vi "Digital Patterns Page.vi"(8 "error in (no error)":errorcluster, 11 "Node Ptr":T1 format="%.0x") -> (0 "error out":errorcluster)   [LabVIEW 2020, in "Engine Simulation Toolkit System Explorer.lvlib"]
uses:
  Engine Simulation Toolkit System Explorer.lvlib
  <vilib>/NI VeriStand/Custom Device API/Custom Device Item Ref.ctl
  Digital Patterns Page Data.ctl
  Digital Pattern.ctl
  Digital Pattern Base.ctl
  Digital Pattern Remove Edge.ctl
  Digital Pattern Add Pulse.ctl
  File Formats.lvlibp/Parent/EST Pattern.ctl
  Shared/Constants and GUIDs.vi
  Shared/Properties.vi
  <vilib>/NI VeriStand/Custom Device API/Custom Device API.lvlib
  Shared/Engine Simulation Toolkit Shared.lvlib
  <vilib>/NI/GXML/GXML.lvlib
  File Formats.lvlibp/Parent/FileFormat.lvclass
panel:
  in  "FPGA Resource":u16(ring) items=["Select an item..."]
  in  "pattern_remove":bool
  in  "pattern_add":bool caption="remove_add"
  in  "add_add":bool caption="remove_add"
  in  "Chart_Offset":dbl caption="Offset" format="%#_6f"
  in  "Chart_Tooth":u16 caption="Tooth"
  in  "Chart_Position":dbl caption="Position" format="%#_6f"
  in  "Edge":bool
  in  "remove_Tooth":u16 caption="Start\nTooth"
  in  "add_Offset":dbl caption="Offset"
  in  "add_Width":dbl caption="Width"
  in  "add_Tooth":u16 caption="Tooth"
  in  "base_Offset":dbl caption="Offset"
  in  "base_Toothwidth":dbl caption="Tooth width"
  in  "base_teeth":u16 caption="Teeth"
  in  "base_Length":dbl caption="Length"
  in  "add_remove":bool
  in  "remove_remove":bool
  in  "remove_add":bool
  in  "Pattern Name":string caption="Name"
  in  "Edges Removed":i32(listbox)
  in  "Pulses Added":i32(listbox)
  in  "Patterns":i32[](listbox)
  in  "Zoom":cluster{dbl, dbl}(slide)={360.0, -360.0} scale=-360.0..360.0
  out "Pattern Plot":cluster{dbl[], dbl[]}[](graph)
  in  "Header":cluster{"Section Name":string}={"Section Name"="Digital Patterns Settings"}
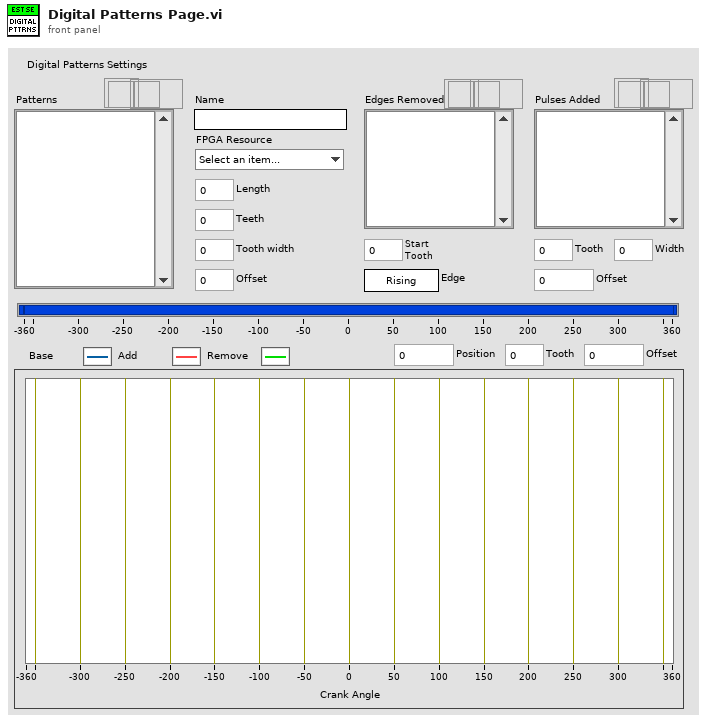
[diagram p1: front panel]
types:
  T1 = typedef "Custom Device API.lvlib/Custom Device Item Ref.ctl" = u64
  T2 = typedef "Engine Simulation Toolkit System Explorer.lvlib/Digital Patterns Page Data.ctl" = cluster{"SysExp Event":refnum<event-registration>, "Init done":bool, "Node Ptr":T1, "Ctrl Refs":cluster{"Header":refnum<vi>, "Pattern Plot":refnum<vi>, "Zoom":refnum<vi>, "Select Pattern":refnum<vi>, "Add List":refnum<vi>, "Remove List":refnum<vi>, "Pattern Name":refnum<vi>, "remove_add":refnum<vi>, "remove_remove":refnum<vi>, "add_remove":refnum<vi>, "base_Length":refnum<vi>, "base_teeth":refnum<vi>, "base_Toothwidth":refnum<vi>, "base_Offset":refnum<vi>, "add_Tooth":refnum<vi>, "add_Width":refnum<vi>, "add_Offset":refnum<vi>, "remove_Tooth":refnum<vi>, "remove_Edge":refnum<vi>, "Chart_Position":refnum<vi>, "Chart_Tooth":refnum<vi>, "Chart_Offset":refnum<vi>, "add_add":refnum<vi>, "pattern_remove":refnum<vi>, "pattern_add":refnum<vi>, "FPGA Resource":refnum<vi>}, "SE ref":refnum<vi>, "Patterns":T3[], "Sel patterns":i32[], "rotations":u16, "Need save":bool, "Rem List":i32, "Add List":i32, "FPGA Resources":string[]}
  T3 = typedef "Engine Simulation Toolkit System Explorer.lvlib/Digital Pattern.ctl" = cluster{"Name":string, "Base":T4, "Remove":T5[], "Add":T6[], "FPGA Resource":string}
  T4 = typedef "Engine Simulation Toolkit System Explorer.lvlib/Digital Pattern Base.ctl" = cluster{"Length":dbl, "Teeth":u16, "Width":dbl, "Offset":dbl}
  T5 = typedef "Engine Simulation Toolkit System Explorer.lvlib/Digital Pattern Remove Edge.ctl" = cluster{"Tooth":u16, "Edge":bool}
  T6 = typedef "Engine Simulation Toolkit System Explorer.lvlib/Digital Pattern Add Pulse.ctl" = cluster{"Tooth":u16, "Offset":dbl, "Width":dbl}
  T7 = typedef "Custom Device API.lvlib/Custom Device Commands.ctl" = enum16{"Default", "Item renamed", "Shutdown", "Dynamic button pressed"}
  T8 = typedef "LVPoint32TypeDef.ctl" = cluster{"Horizontal":i32, "Vertical":i32}
  T9 = typedef "File Formats.lvlibp/FileFormat.lvclass/EST Pattern.ctl" = cluster{"Base":cluster{"Length":dbl, "Teeth":u16, "Width":dbl, "Offset":dbl}, "Remove":cluster{"Tooth":u16, "Edge":bool}[], "Add":cluster{"Tooth":u16, "Offset":dbl, "Width":dbl}[]}
  T10 = cluster{"Length":dbl, "Teeth":u16, "Width":dbl, "Offset":dbl}
  T11 = cluster{"Tooth":u16, "Offset":dbl, "Width":dbl}[]
  T12 = cluster{"ip list property name":string, string[]}[]
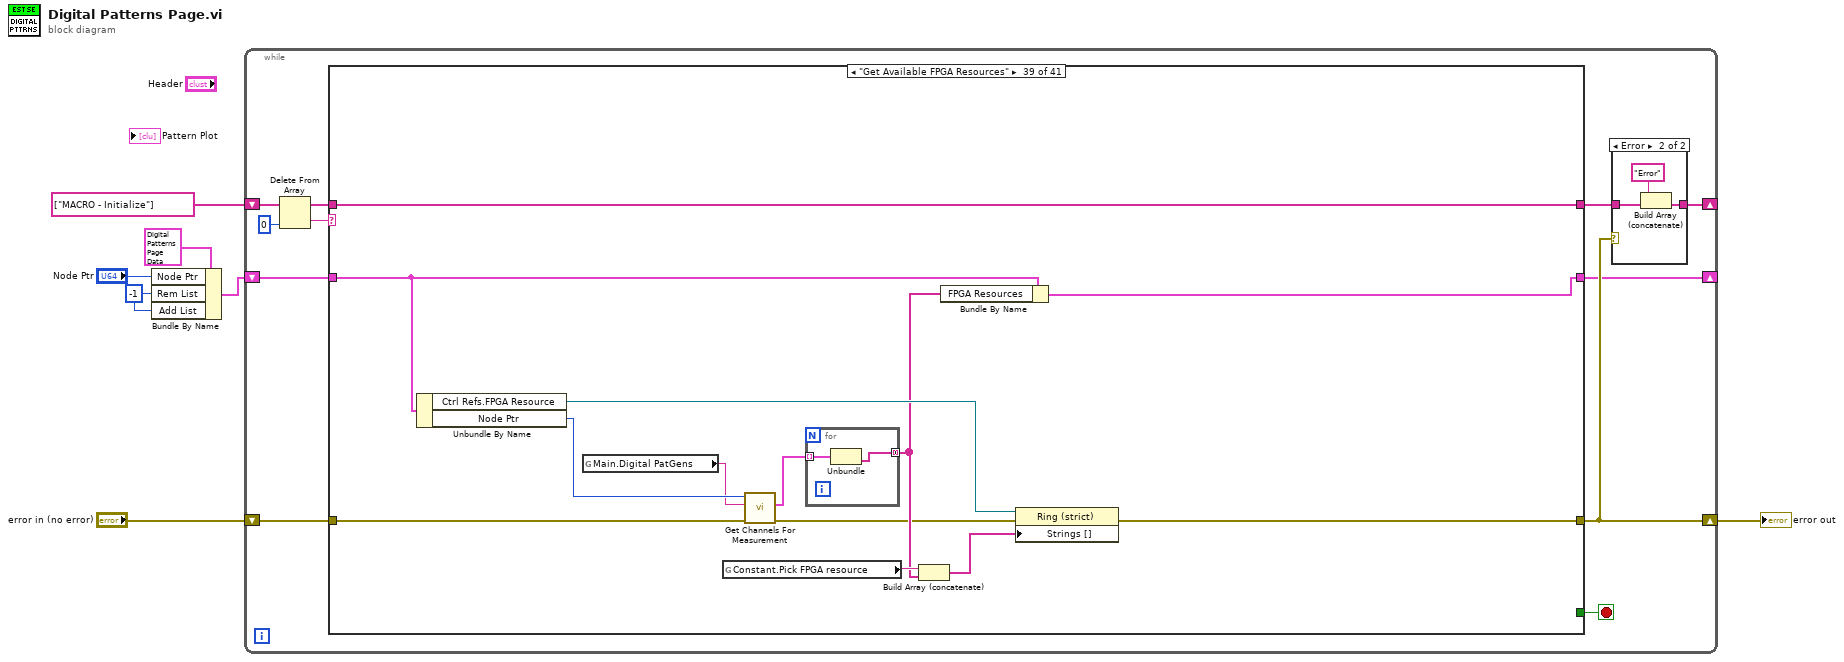
[diagram p0: block diagram]
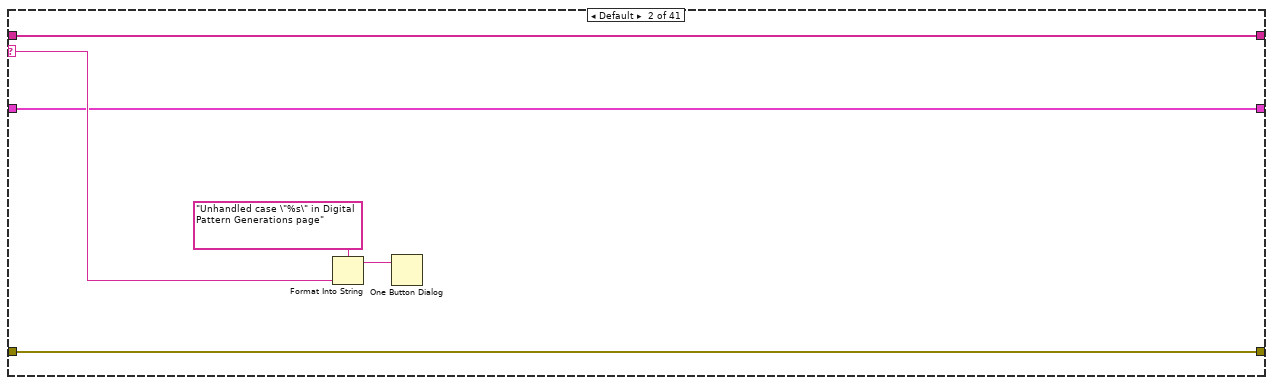
[diagram p4: hidden frame]
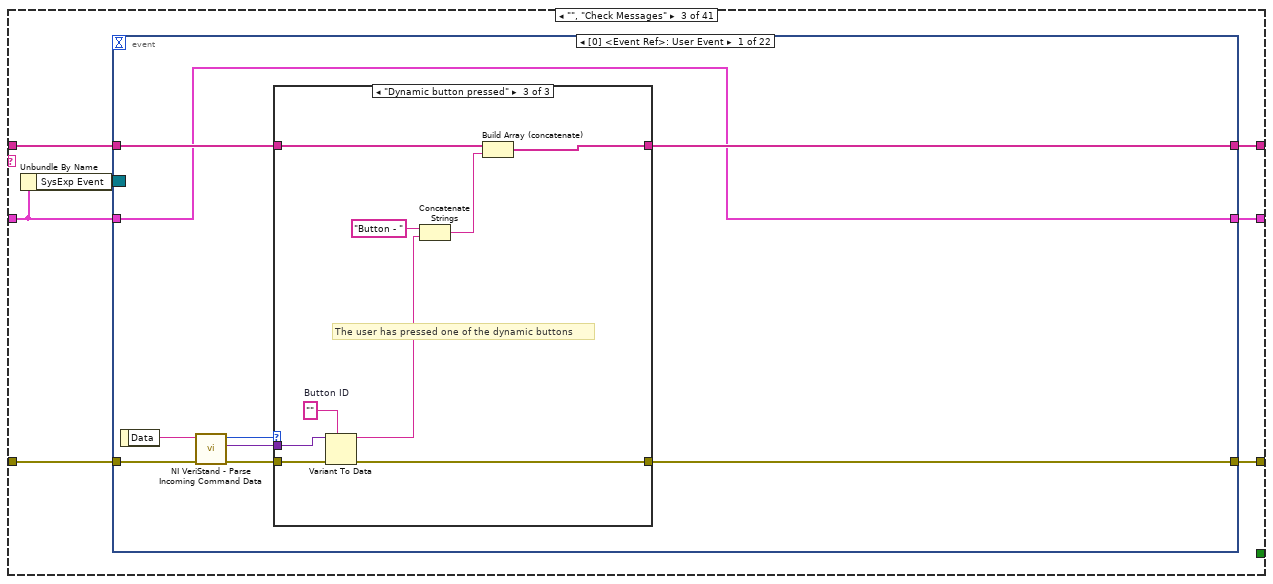
[diagram p5: hidden frame]
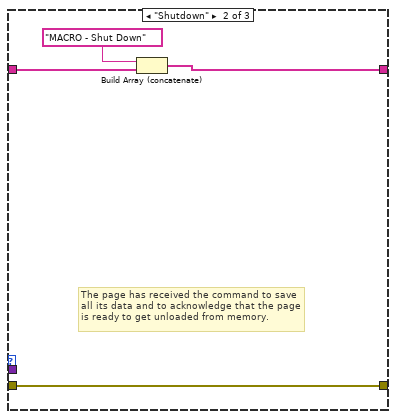
[diagram p7: hidden frame]
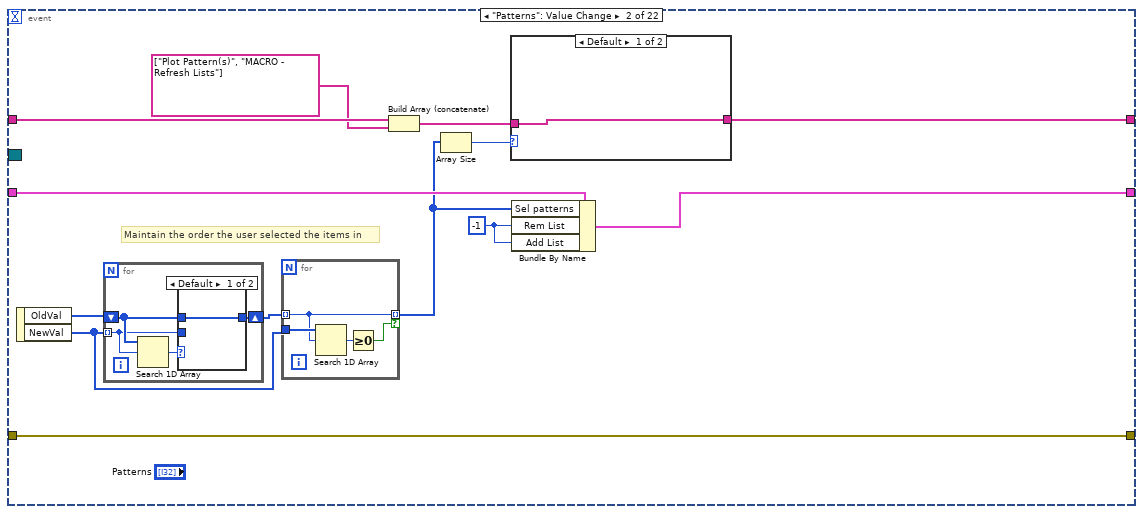
[diagram p8: hidden frame]
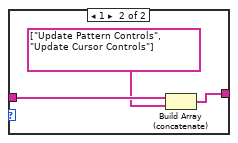
[diagram p9: hidden frame]
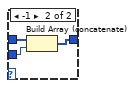
[diagram p10: hidden frame]
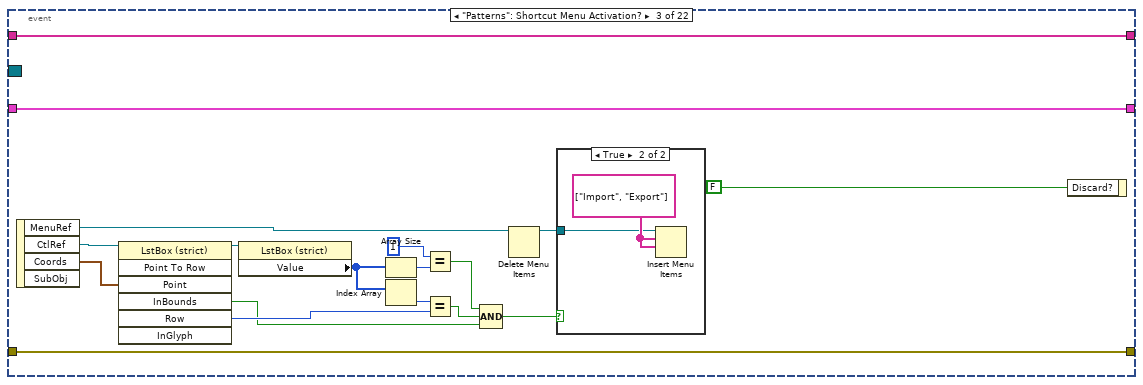
[diagram p11: hidden frame]
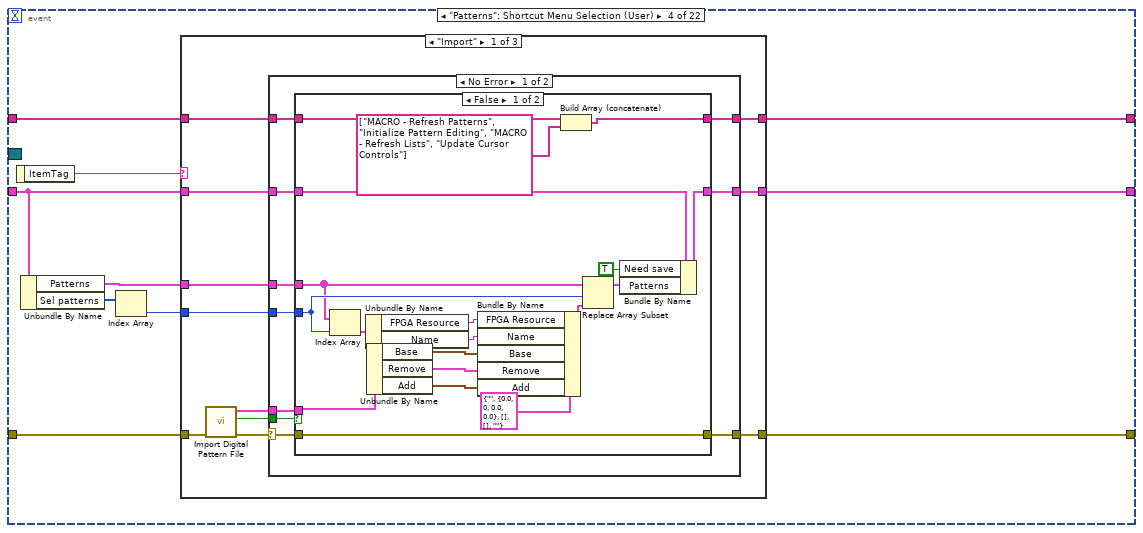
[diagram p13: hidden frame]
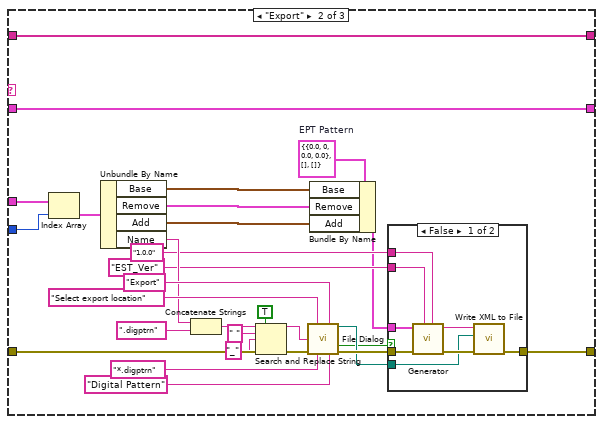
[diagram p16: hidden frame]
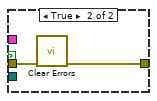
[diagram p17: hidden frame]
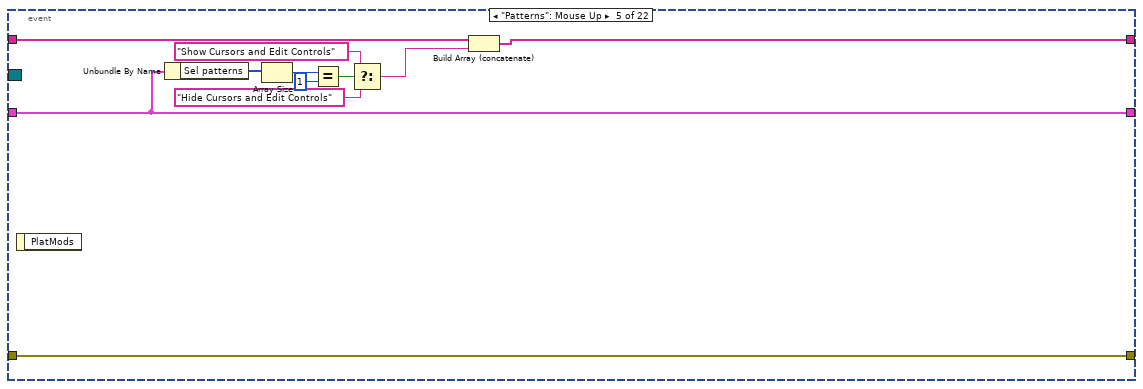
[diagram p19: hidden frame]
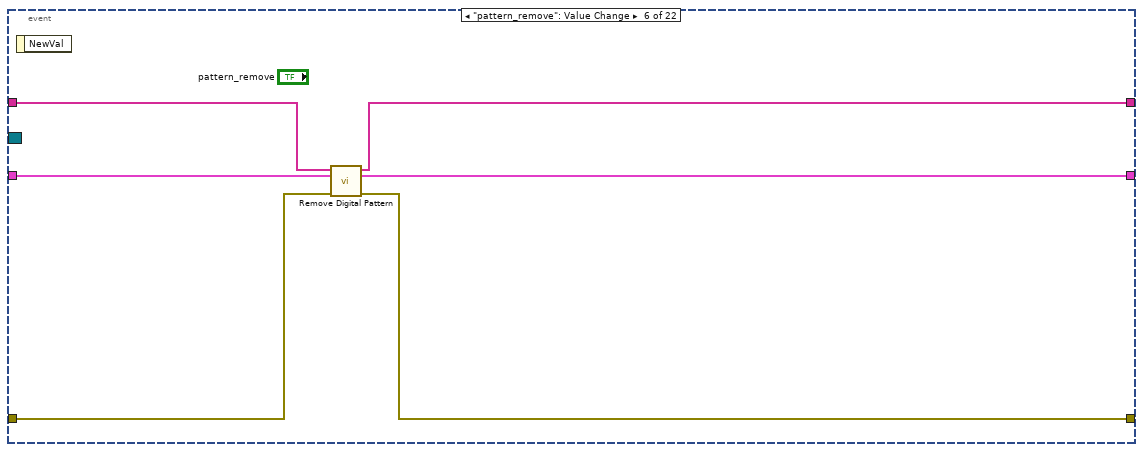
[diagram p20: hidden frame]
diagram:
  w1 = -1 ("Rem List")
  n1 = Bundle By Name(cluster=T2 {"SysExp Event"=refnum, "Init done"=FALSE, "Node Ptr"=0, "Ctrl Refs"={"Header"=refnum, "Pattern Plot"=refnum, "Zoom"=refnum, "Select Pattern"=refnum, "Add List"=refnum, "Remove List"=refnum, "Pattern Name"=refnum, "remove_add"=refnum, "remove_remove"=refnum, "add_remove"=refnum, "base_Length"=refnum, "base_teeth"=refnum, "base_Toothwidth"=refnum, "base_Offset"=refnum, "add_Tooth"=refnum, "add_Width"=refnum, "add_Offset"=refnum, "remove_Tooth"=refnum, "remove_Edge"=refnum, "Chart_Position"=refnum, "Chart_Tooth"=refnum, "Chart_Offset"=refnum, "add_add"=refnum, "pattern_remove"=refnum, "pattern_add"=refnum, "FPGA Resource"=refnum}, "SE ref"=refnum, "Patterns"=[], "Sel patterns"=[], "rotations"=0, "Need save"=FALSE, "Rem List"=0, "Add List"=0, "FPGA Resources"=[]} ("Page Data"), "Node Ptr"="Node Ptr", "Rem List"=w1, "Add List"=w1) -> (w3:T2)
  n2 = while {
    shift-right: [w13] -> _
    shift-left: string[] ["MACRO - Initialize"] -> [w18]
    shift-right: [w10] -> w5
    shift-left: "error in (no error)" -> [w12]
    shift-right: [w9] -> _
    shift-left: w3 -> [w14]
    stop <- w16 stop-if-true
    n3 = Delete From Array(array=w18, index=0) -> (deleted portion=w8:string, array with subset deleted=w17:string[])  [unwired: 1 in]
    n4 = case shown="\"Get Available FPGA Resources\"" w8 {
      selector: w8 -> [_ w30 _ _ _ _ _ _ _ _ _ _ _ _ _ _ _ _ _ _ _ _ _ _ _ _ _ _ _ _ _ _ _ _ _ _ _ _ _ _ _]
      tunnel: [w23 w26 w38 w543 w557 w561 w564 w580 w589 w594 w598 w609 w627 w638 w650 w662 w666 w703 w760 w785 w800 w801 w810 w826 w827 w831 w834 w841 w846 w851 w854 w884 w890 w898 w905 w910 w917 w933 w946 w955 w960] -> w15
      tunnel: w17 -> [w23 w26 w37 w544 w557 w561 w564 w580 w589 w594 w598 w609 w627 w638 w650 w662 w673 w706 w760 w785 w800 w801 w810 w826 w827 w831 w835 w842 w847 w852 w854 w884 w890 w898 w905 w910 w917 w933 w946 w955 w961]
      tunnel: [_ _ _ _ _ _ _ _ _ _ _ _ _ _ _ _ _ _ _ _ _ _ _ _ TRUE _ _ _ _ _ _ _ _ _ _ _ _ _ _ _ _] -> w16
      tunnel: w12 -> [w25 w28 w35 w548 w556 w560 w563 w567 w588 w593 w597 w608 w626 w637 w649 w661 w669 w705 w759 w784 w799 w803 w809 w821 w829 w833 w838 w843 w848 w853 w856 w883 w888 w895 w902 w909 w916 w932 w938 w954 w957]
      tunnel: [w25 w28 w32 errorcluster {"status"=FALSE, "code"=0, "source"=""} ("error constant") w555 w560 w563 w567 w587 w591 w596 w603 w626 w637 w649 w661 w668 w704 w759 w784 w799 w803 w807 w822 w829 w833 w838 w843 w848 w853 w856 w883 w887 w894 w901 w909 w912 w921 w943 w954 w957] -> w10
      tunnel: w14 -> [w24 w27 w34 w546 w554 w559 w562 w570 w586 w590 w595 w607 w625 w636 w648 w660 w667 w700 w758 w783 w798 w802 w808 w825 w828 w832 w837 w840 w845 w850 w855 w886 w889 w893 w904 w908 w915 w931 w945 w953 w958]
      tunnel: [w24 w27 w36 w546 w554 w559 w562 w570 w586 w590 w595 w600 w625 w636 w648 w660 w667 w700 w758 w783 w798 w802 w808 w825 w828 w832 w837 w840 w845 w850 w855 w885 w889 w891 w900 w907 w913 w930 w944 w951 w958] -> w9
      frame "<------------------ System ------------------>" {
      }
      frame Default {
        n5 = Format Into String(format string="Unhandled case \"%s\" in Digital Pattern Generations page", w30) -> (resulting string=w31:string)  [unwired: 2 in, 1 out]
        n6 = One Button Dialog(message=w31) -> ()  [unwired: 1 in, 1 out]
      }
      frame "", "Check Messages" {
        n7 = Unbundle By Name(w34) -> ("SysExp Event"=w33:refnum<event-registration>)
        n8 = event shown="[0] <Event Ref>: User Event" {
          selector: w33 -> [_ _ _ _ _ _ _ _ _ _ _ _ _ _ _ _ _ _ _ _ _ _]
          dyn-events: _ -> [_ _ _ _ _ _ _ _ _ _ _ _ _ _ _ _ _ _ _ _ _ _]
          timeout: _ -> [_ _ _ _ _ _ _ _ _ _ _ _ _ _ _ _ _ _ _ _ _ _]
          tunnel: [w40 w66 w109 w113 w213 w223 w229 w242 w250 w267 w291 w353 w375 w388 w396 w419 w434 w442 w446 w466 w494 w531] -> w38
          tunnel: w37 -> [w41 w75 w109 w112 w214 w226 w232 w242 w260 w262 w292 w361 w383 w389 w397 w420 w435 w443 w463 w483 w505 w542]
          tunnel: [w39 w70 w108 w117 w219 w224 w230 w241 w252 w268 w293 w355 w377 w386 w395 w418 w430 w438 w449 w469 w496 w533] -> w36
          tunnel: w34 -> [w39 w74 w108 w116 w219 w225 w231 w241 w253 w269 w299 w356 w378 w391 w415 w427 w432 w440 w461 w481 w503 w540]
          tunnel: w35 -> [w47 w69 w107 w115 w220 w222 w228 w240 w259 w263 w294 w360 w382 w390 w413 w425 w431 w439 w462 w482 w504 w541]
          tunnel: [w42 w69 w107 w114 w220 w221 w227 w239 w259 w264 w295 w360 w382 w390 w399 w422 w431 w439 w462 w482 w504 w541] -> w32
          event User Event {
            n9 = event-data() -> ("Data"=w46:string)  [unwired: 1 in]
            n10 = call <vilib>:"NI VeriStand - Parse Incoming Command Data.vi"("error in (no error)"=w47, "Incoming data"=w46) -> ("error out"=w44:errorcluster, "Outgoing data"=w43:variant, "Action"=w45:T7)  [unwired: 7 out]
            n11 = case shown="\"Dynamic button pressed\"" w45 {
              tunnel: [w49 w53 w61] -> w42
              tunnel: w44 -> [w49 w53 w60]
              tunnel: w43 -> [_ _ w59]
              tunnel: w41 -> [w48 w52 w58]
              tunnel: [w48 w50 w57] -> w40
              frame "Default", Default {
              }
              frame "Shutdown" {
                # "The page has received the command to save all its data and to acknowledge that the page is ready to get unloaded from memory."
                n12 = Build Array (concatenate)("MACRO - Shut Down", w52) -> (w50:string[])
              }
              frame "Dynamic button pressed" {
                w62 = ""  # Button ID
                # "The user has pressed one of the dynamic buttons"
                n13 = Variant To Data(error in=w60, type=w62, Variant=w59) -> (data=w55:string, error out=w61:errorcluster)
                n14 = Concatenate Strings("Button - " ("string"), w55) -> (w54:string)
                n15 = Build Array (concatenate)(w58, w54) -> (w57:string[])
              }
            }
          }
          event "Patterns": Value Change {
            w63 = -1 ("Rem List")
            # "Maintain the order the user selected the items in"
            n16 = event-data() -> ("OldVal"=w71:i32[], "NewVal"=w72:i32[])  [unwired: 1 in]
            n17 = for {
              tunnel: w72 -> [w84] mode=indexing
              shift-right: [w85] -> w73
              shift-left: w71 -> [w86]
              n18 = Search 1D Array(1D array=w86, element=w84) -> (index of element=w87:i32)  [unwired: 1 in]
              n19 = case shown="Default" w87 {
                tunnel: w86 -> [w88 w91]
                tunnel: [w88 w90] -> w85
                tunnel: w84 -> [_ w89]
                frame Default {
                }
                frame -1 {
                  n20 = Build Array (concatenate)(w91, w89) -> (w90:i32[])
                }
              }
            }
            n21 = for {
              tunnel: w72 -> [w81]
              tunnel: w73 -> [w80] mode=indexing
              tunnel: [w80] -> w65 mode=indexing if=w82
              n22 = Search 1D Array(1D array=w81, element=w80) -> (index of element=w83:i32)  [unwired: 1 in]
              n23 = Greater Or Equal To 0?(x=w83) -> (x >= 0?=w82:bool)
            }
            n24 = Build Array (concatenate)(w75, string[] ["Plot Pattern(s)", "MACRO - Refresh Lists"]) -> (w68:string[])
            n25 = Array Size(array=w65) -> (size(s)=w64:i32)
            n26 = case shown="Default" w64 {
              tunnel: w68 -> [w76 w79]
              tunnel: [w76 w78] -> w66
              frame Default {
              }
              frame 1 {
                n27 = Build Array (concatenate)(w79, string[] ["Update Pattern Controls", "Update Cursor Controls"]) -> (w78:string[])
              }
            }
            n28 = Bundle By Name(cluster=w74, "Sel patterns"=w65, "Rem List"=w63, "Add List"=w63) -> (w70:T2)
          }
          event "Patterns": Shortcut Menu Activation? {
            n29 = event-data() -> ("MenuRef"=w93:refnum<k9>, "CtlRef"=w105:refnum<vi>, "Coords"=w106:T8)  [unwired: 1 in, 1 out]
            n30 = invoke class="LstBox (strict)" method="Point To Row"(reference=w105, "Point"=w106) -> (reference out=w104:refnum<vi>, "InBounds"=w97:bool, "Row"=w98:i32)  [unwired: 5 in, 4 out]
            n31 = property class="LstBox (strict)"(reference=w104) -> ("Value"=w102:i32[])  [unwired: 1 in, 2 out]
            n32 = Array Size(array=w102) -> (size(s)=w101:i32)
            n33 = Index Array(array=w102) -> (element=w99:i32)  [unwired: 1 in]
            n34 = Equal?(x=1 ("y"), y=w101) -> (x = y?=w95:bool)
            n35 = Equal?(x=w99, y=w98) -> (x = y?=w96:bool)
            n36 = Compound Arithmetic op=AND(w95, w96, w97) -> (w94:bool)
            n37 = Delete Menu Items(9:w93) -> (3:w92:refnum<k9>)  [unwired: 3 in, 1 out]
            n38 = case shown="True" w94 {
              tunnel: w92 -> [_ w110]
              frame False {
              }
              frame True {
                w111 = string[] ["Import", "Export"] ("item names")
                n39 = Insert Menu Items(7:w111, 8:w111, 9:w110) -> ()  [unwired: 3 in, 3 out]
              }
            }
            n40 = event-data("Discard?"=FALSE) -> ()  [unwired: 1 in, 1 out]
          }
          event "Patterns": Shortcut Menu Selection (User) {
            n41 = event-data() -> ("ItemTag"=w118:string)  [unwired: 1 in]
            n42 = Unbundle By Name(w116) -> ("Patterns"=w119:T3[], "Sel patterns"=w120:i32[])
            n43 = Index Array(array=w120) -> (element=w121:i32)  [unwired: 1 in]
            n44 = case shown="\"Import\"" w118 {
              tunnel: w121 -> [w130 w196 _]
              tunnel: w119 -> [w123 w195 _]
              tunnel: [w131 w194 w209] -> w117
              tunnel: w116 -> [w132 w194 w209]
              tunnel: w115 -> [w126 w175 w208]
              tunnel: [w129 w193 w208] -> w114
              tunnel: [w128 w185 w207] -> w113
              tunnel: w112 -> [w127 w185 w207]
              frame "Import" {
                n45 = call "Import Digital Pattern File.vi"("error in (no error)"=w126) -> ("error out"=w122:errorcluster, "Canceled?"=w125:bool, "EPT Pattern"=w124:T9)  [unwired: 8 in]
                n46 = case shown="No Error" w122 {
                  selector: w122 -> [w133 w167]
                  tunnel: w132 -> [w142 w166]
                  tunnel: [w141 w166] -> w131
                  tunnel: w130 -> [w140 _]
                  tunnel: [w139 w167] -> w129
                  tunnel: [w138 w165] -> w128
                  tunnel: w127 -> [w137 w165]
                  tunnel: w125 -> [w136 _]
                  tunnel: w124 -> [w135 _]
                  tunnel: w123 -> [w134 _]
                  frame No Error {
                    n47 = case shown="False" w136 {
                      tunnel: w142 -> [w161 w164]
                      tunnel: [w160 w164] -> w141
                      tunnel: w134 -> [w151 _]
                      tunnel: w140 -> [w152 _]
                      tunnel: w133 -> [w159 w162]
                      tunnel: [w159 w162] -> w139
                      tunnel: [w158 w163] -> w138
                      tunnel: w137 -> [w157 w163]
                      tunnel: w135 -> [w150 _]
                      frame False {
                        n48 = Index Array(array=w151, index=w152) -> (element=w155:T3)
                        n49 = Unbundle By Name(w155) -> ("FPGA Resource"=w154:string, "Name"=w153:string)
                        n50 = Unbundle By Name(w150) -> ("Base"=w145:T10, "Remove"=w144:cluster{"Tooth":u16, "Edge":bool}[], "Add"=w143:T11)
                        n51 = Bundle By Name(cluster=T3 {"Name"="", "Base"={"Length"=0.0, "Teeth"=0, "Width"=0.0, "Offset"=0.0}, "Remove"=[], "Add"=[], "FPGA Resource"=""} ("element"), "FPGA Resource"=w154, "Name"=w153, "Base"=w145, "Remove"=w144, "Add"=w143) -> (w147:T3)
                        n52 = Build Array (concatenate)(w157, string[] ["MACRO - Refresh Patterns", "Initialize Pattern Editing", "MACRO - Refresh Lists", "Update Cursor Controls"]) -> (w158:string[])
                        n53 = Replace Array Subset(array=w151, new element=w147, index=w152) -> (w149:T3[])
                        n54 = Bundle By Name(cluster=w161, "Need save"=TRUE, "Patterns"=w149) -> (w160:T2)
                      }
                      frame True {
                      }
                    }
                  }
                  frame Error {
                  }
                }
              }
              frame "Export" {
                w168 = T9 {"Base"={"Length"=0.0, "Teeth"=0, "Width"=0.0, "Offset"=0.0}, "Remove"=[], "Add"=[]}  # EPT Pattern
                n55 = Index Array(array=w195, index=w196) -> (element=w187:T3)
                n56 = Unbundle By Name(w187) -> ("Base"=w179:T4, "Remove"=w178:T5[], "Add"=w177:T6[], "Name"=w186:string)
                n57 = Concatenate Strings(w186, ".digptrn" ("button label")) -> (w172:string)
                n58 = Search and Replace String(replace all?=TRUE ("replace all? (F)"), input string=w172, search string=" ", replace string="_" ("replace string (\"\")"), error in=w175) -> (result string=w173:string, error out=w174:errorcluster)  [unwired: 3 in, 2 out]
                n59 = call "File Dialog"("prompt"="Select export location", "button label"="Export", "default name"=w173, "error in"=w174, "pattern (all files)"="*.digptrn" ("button label"), "pattern label"="Digital Pattern" ("button label")) -> ("selected path"=w190:path, "cancelled"=w189:bool, "error out"=w192:errorcluster)  [unwired: 6 in, 1 out]
                n60 = Bundle By Name(cluster=w168, "Base"=w179, "Remove"=w178, "Add"=w177) -> (w176:T9)
                n61 = case shown="False" w189 {
                  tunnel: w176 -> [w204 _]
                  tunnel: [w201 w205] -> w193
                  tunnel: w192 -> [w200 w206]
                  tunnel: w190 -> [w199 _]
                  tunnel: "EST_Ver" ("prompt") -> [w198 _]
                  tunnel: "1.0.0" ("button label") -> [w197 _]
                  frame False {
                    n62 = call <vilib>:"Generator.vi"("Version String"=w197, "Version Tag Name"=w198, "error in"=w200, "Variant"=w204) -> ("error out"=w202:errorcluster, "XML String Out"=w203:string)  [unwired: 6 in]
                    n63 = call <vilib>:"Write XML to File.vi"("error in"=w202, "XML File Path"=w199, "XML Input"=w203) -> ("error out"=w201:errorcluster)  [unwired: 8 in]
                  }
                  frame True {
                    n64 = call <vilib>:"Clear Errors.vi"("error in (no error)"=w206) -> ("error out"=w205:errorcluster)  [unwired: 5 in, 1 out]
                  }
                }
              }
              frame Default {
              }
            }
          }
          event "Patterns": Mouse Up {
            n65 = event-data() -> ()  [unwired: 1 in, 1 out]
            n66 = Unbundle By Name(w219) -> ("Sel patterns"=w218:i32[])
            n67 = Array Size(array=w218) -> (size(s)=w217:i32)
            n68 = Equal?(x=w217, y=1) -> (x = y?=w215:bool)
            n69 = Select(t="Show Cursors and Edit Controls", s=w215, f="Hide Cursors and Edit Controls") -> (s? t:f=w210:string)
            n70 = Build Array (concatenate)(w214, w210) -> (w213:string[])
          }
          event "pattern_remove": Value Change {
            n71 = event-data() -> ()  [unwired: 1 in, 1 out]
            n72 = call "Remove Digital Pattern.vi"("error in (no error)"=w222, "Page Data in"=w225, "State queue in"=w226) -> ("error out"=w221:errorcluster, "Page Data out"=w224:T2, "State queue out"=w223:string[])  [unwired: 6 in]
          }
          event "pattern_add": Value Change {
            n73 = event-data() -> ()  [unwired: 1 in, 1 out]
            n74 = call "Add Digital Pattern.vi"("error in (no error)"=w228, "Page Data in"=w231, "State queue in"=w232) -> ("error out"=w227:errorcluster, "Page Data out"=w230:T2, "State queue out"=w229:string[])  [unwired: 6 in]
          }
          event "Zoom": Value Change {
            n75 = event-data() -> ("NewVal"=w235:cluster{dbl, dbl})  [unwired: 1 in]
            n76 = Unbundle By Name(w241) -> ("Ctrl Refs.Pattern Plot"=w238:refnum<vi>)
            n77 = Unbundle(w235) -> (w237:dbl, w236:dbl)
            n78 = Max & Min(x=w237, y=w236) -> (max(x,y)=w234:dbl, min(x,y)=w233:dbl)
            n79 = property on="Property Node" class="XYGraph (strict)"(reference=w238, error in=w240, "XScale.Maximum"=w234, "XScale.Minimum"=w233) -> (error out=w239:errorcluster)  [unwired: 1 out]
          }
          event "base_Length", "base_teeth", "base_Toothwidth", "base_Offset": Value Change {
            n80 = event-data() -> ()  [unwired: 1 in, 6 out]
            n81 = Unbundle By Name(w253) -> ("Patterns"=w255:T3[], "Sel patterns"=w254:i32[])
            n82 = Index Array(array=w254) -> (element=w256:i32)  [unwired: 1 in]
            n83 = Build Array (concatenate)(w260, "Plot Pattern(s)", "Update Cursor Controls") -> (w250:string[])
            n84 = Index Array(array=w255, index=w256) -> (element=w257:T3)
            n85 = Bundle By Name(cluster=w257, "Base.Length"="base_Length", "Base.Teeth"="base_teeth", "Base.Width"="base_Toothwidth", "Base.Offset"="base_Offset") -> (w258:T3)
            n86 = Replace Array Subset(array=w255, new element=w258, index=w256) -> (w251:T3[])
            n87 = Bundle By Name(cluster=w253, "Patterns"=w251, "Need save"=TRUE) -> (w252:T2)
          }
          event "Pattern Name": Value Change {
            n88 = event-data() -> ("NewVal"=w265:string, "OldVal"=w266:string)  [unwired: 1 in]
            n89 = call "Rename Digital Pattern.vi"("OldVal"=w266, "error in (no error)"=w263, "NewVal"=w265, "Page Data in"=w269, "State Queue in"=w262) -> ("error out"=w264:errorcluster, "name collision?"=w261:bool, "Page Data out"=w268:T2, "State Queue out"=w267:string[])  [unwired: 3 in]
            n90 = case shown="True" w261 {
              frame False {
              }
              frame True {
                n91 = One Button Dialog(message="Could not change Name due to a naming conflict.") -> ()  [unwired: 1 in, 1 out]
              }
            }
          }
          event "FPGA Resource": Value Change {
            n92 = event-data() -> ("OldVal"=w272:u16, "NewVal"=w289:u16)  [unwired: 1 in]
            n93 = Unbundle By Name(w299) -> ("Node Ptr"=w288:T1, "Patterns"=w278:T3[], "Sel patterns"=w298:i32[], "FPGA Resources"=w297:string[])
            n94 = Decrement(x=w272) -> (x-1=w296:u16)
            n95 = Decrement(x=w289) -> (x-1=w290:u16)
            n96 = Index Array(array=w297, index #1=w296, index #2=w290) -> (element #1=w286:string, element #2=w285:string)
            n97 = Index Array(array=w298) -> (element=w287:i32)  [unwired: 1 in]
            n98 = Index Array(array=w278, index=w287) -> (element=w283:T3)
            n99 = call "Get RIO and Channel Strings.vi"("rio/channel"=w285) -> ("channel"=w279:string, "rio"=w274:string)  [unwired: 9 in]
            n100 = call "Get RIO and Channel Strings.vi"("rio/channel"=w286) -> ("channel"=w282:string, "rio"=w273:string)  [unwired: 9 in]
            n101 = Unbundle By Name(w283) -> ("Name"=w271:string)
            n102 = Equal?(x=w271, y=w282) -> (x = y?=w281:bool)
            n103 = Not Equal To 0?(x=w289) -> (x != 0?=w284:bool)
            n104 = And(x=w281, y=w284) -> (x .and. y?=w280:bool)
            n105 = Select(t=w279, s=w280, f=w271) -> (s? t:f=w277:string)
            n106 = call "Check Digital Pattern Name Collisions.vi"("old name"=w271, "old rio"=w273, "new name"=w277, "new rio"=w274, "Patterns"=w278) -> ("name collision?"=w275:bool, "Patterns"=w276:T3[])  [unwired: 5 in]
            n107 = case shown="False" w275 {
              tunnel: w299 -> [w317 w340]
              tunnel: [w316 w338] -> w295
              tunnel: w294 -> [w315 w338]
              tunnel: [w314 w340] -> w293
              tunnel: w292 -> [w313 w339]
              tunnel: [w312 w339] -> w291
              tunnel: w288 -> [w311 _]
              tunnel: w287 -> [w310 _]
              tunnel: w286 -> [w309 _]
              tunnel: w285 -> [w308 _]
              tunnel: w283 -> [w304 _]
              tunnel: w280 -> [w302 _]
              tunnel: w271 -> [w301 _]
              tunnel: w276 -> [w300 _]
              tunnel: w272 -> [_ w337]
              frame False {
                n108 = Bundle By Name(cluster=w304, "FPGA Resource"=w308) -> (w303:T3)
                n109 = Replace Array Subset(array=w300, new element=w303, index=w310) -> (w305:T3[])
                n110 = Bundle By Name(cluster=w317, "Patterns"=w305, "Need save"=TRUE) -> (w306:T2)
                n111 = case shown="False" w302 {
                  tunnel: [w324 w334] -> w316
                  tunnel: w315 -> [w325 w335]
                  tunnel: w309 -> [w318 w333]
                  tunnel: w308 -> [w322 w332]
                  tunnel: w306 -> [w326 w331]
                  tunnel: [w326 w330] -> w314
                  tunnel: w313 -> [w327 w329]
                  tunnel: [w327 w328] -> w312
                  tunnel: w301 -> [w323 _]
                  tunnel: w311 -> [w320 _]
                  frame False {
                    n112 = call "Get RIO and Channel Strings.vi"("rio/channel"=w318) -> ("rio"=w319:string)  [unwired: 9 in, 1 out]
                    n113 = call "Get RIO and Channel Strings.vi"("rio/channel"=w322) -> ("rio"=w321:string)  [unwired: 9 in, 1 out]
                    n114 = call "Move Digital Pattern to RIO.vi"("New RIO"=w321, "error in (no error)"=w325, "Name"=w323, "Old RIO"=w319, "Item Ref in"=w320) -> ("error out"=w324:errorcluster)  [unwired: 4 in, 2 out]
                  }
                  frame True {
                    n115 = call "Rename Digital Pattern From FPGA Resource.vi"("Old FPGA Resource"=w333, "error in (no error)"=w335, "New FPGA Resource"=w332, "Page Data in"=w331, "State Queue in"=w329) -> ("error out"=w334:errorcluster, "Page Data out"=w330:T2, "State Queue out"=w328:string[])  [unwired: 4 in]
                  }
                }
              }
              frame True {
                n116 = local write "FPGA Resource"(w337) -> ()
                n117 = One Button Dialog(message="Could not change FPGA Resource due to a naming conflict.") -> ()  [unwired: 1 in, 1 out]
              }
            }
          }
          event "remove_Tooth", "Edge": Value Change {
            # "internally teeth are zero indexed, but they are 1 indexed on GUI"
            n118 = event-data() -> ()  [unwired: 1 in, 1 out]
            n119 = Unbundle By Name(w356) -> ("Patterns"=w358:T3[], "Sel patterns"=w357:i32[], "Rem List"=w350:i32)
            n120 = Index Array(array=w357) -> (element=w359:i32)  [unwired: 1 in]
            n121 = Decrement(x="remove_Tooth") -> (x-1=w341:u16)
            n122 = Index Array(array=w358, index=w359) -> (element=w344:T3)
            n123 = Bundle By Name(cluster=T5 {"Tooth"=0, "Edge"=FALSE} ("Cluster"), "Tooth"=w341, "Edge"="Edge") -> (w346:T5)
            n124 = Unbundle By Name(w344) -> ("Remove"=w351:T5[])
            n125 = Replace Array Subset(array=w351, new element=w346, index=w350) -> (w345:T5[])
            n126 = Build Array (concatenate)(w361, string[] ["Refresh Remove List", "MACRO - Refresh Patterns", "Update Pattern Controls"]) -> (w353:string[])
            n127 = Bundle By Name(cluster=w344, "Remove"=w345) -> (w343:T3)
            n128 = Replace Array Subset(array=w358, new element=w343, index=w359) -> (w354:T3[])
            n129 = Bundle By Name(cluster=w356, "Patterns"=w354, "Need save"=TRUE) -> (w355:T2)
          }
          event "add_Tooth", "add_Width", "add_Offset": Value Change {
            # "internally teeth are zero indexed, but they are 1 indexed on GUI"
            n130 = event-data() -> ()  [unwired: 1 in, 3 out]
            n131 = Unbundle By Name(w378) -> ("Patterns"=w380:T3[], "Sel patterns"=w379:i32[], "Add List"=w372:i32)
            n132 = Index Array(array=w379) -> (element=w381:i32)  [unwired: 1 in]
            n133 = Decrement(x="add_Tooth") -> (x-1=w362:u16)
            n134 = Index Array(array=w380, index=w381) -> (element=w368:T3)
            n135 = Bundle By Name(cluster=T6 {"Tooth"=0, "Offset"=0.0, "Width"=0.0} ("Cluster"), "Tooth"=w362, "Offset"="add_Offset", "Width"="add_Width") -> (w370:T6)
            n136 = Unbundle By Name(w368) -> ("Add"=w373:T6[])
            n137 = Replace Array Subset(array=w373, new element=w370, index=w372) -> (w369:T6[])
            n138 = Build Array (concatenate)(w383, string[] ["Refresh Add List", "MACRO - Refresh Patterns", "Update Pattern Controls"]) -> (w375:string[])
            n139 = Bundle By Name(cluster=w368, "Add"=w369) -> (w367:T3)
            n140 = Replace Array Subset(array=w380, new element=w367, index=w381) -> (w376:T3[])
            n141 = Bundle By Name(cluster=w378, "Patterns"=w376, "Need save"=TRUE) -> (w377:T2)
          }
          event "Pattern Plot": Cursor Move {
            w385 = -1 ("Add List")
            n142 = event-data() -> ()  [unwired: 1 in, 1 out]
            n143 = Build Array (concatenate)(w389, "MACRO - Refresh Lists", "Update Cursor Controls") -> (w388:string[])
            n144 = Bundle By Name(cluster=w391, "Rem List"=w385, "Add List"=w385) -> (w386:T2)
          }
          event "Chart_Tooth", "Chart_Offset": Value Change {
            w394 = -1 ("Add List")
            # "internally teeth are zero indexed, but they are 1 indexed on GUI"
            n145 = event-data() -> ()  [unwired: 1 in, 1 out]
            n146 = Unbundle By Name(w415) -> ("Patterns"=w410:T3[], "Sel patterns"=w409:i32[], "Ctrl Refs.Pattern Plot"=w412:refnum<vi>)
            n147 = Index Array(array=w409) -> (element=w411:i32)  [unwired: 1 in]
            n148 = Index Array(array=w410, index=w411) -> (element=w408:T3)
            n149 = Unbundle By Name(w408) -> ("Base.Length"=w404:dbl, "Base.Teeth"=w405:u16, "Base.Offset"=w403:dbl)
            n150 = Decrement(x="Chart_Tooth") -> (x-1=w392:u16)
            n151 = Divide(x=w404, y=w405) -> (x/y=w406:dbl)
            n152 = Multiply(x=w392, y=w406) -> (x*y=w407:dbl)
            n153 = Compound Arithmetic op=ADD(w407, "Chart_Offset", w403) -> (w400:dbl)
            n154 = Build Array (concatenate)(w397, "MACRO - Refresh Lists", "Update Cursor Controls") -> (w396:string[])
            n155 = property on="Property Node" class="XYGraph (strict)"(reference=w412, error in=w413, "Active Cursor"=u32 0, "Cursor.Cursor X"=w400) -> (error out=w399:errorcluster)  [unwired: 1 out]
            n156 = Bundle By Name(cluster=w415, "Rem List"=w394, "Add List"=w394) -> (w395:T2)
          }
          event "Chart_Position": Value Change {
            w417 = -1 ("Add List")
            n157 = event-data() -> ("NewVal"=w423:dbl)  [unwired: 1 in]
            n158 = Unbundle By Name(w427) -> ("Ctrl Refs.Pattern Plot"=w424:refnum<vi>)
            n159 = property on="Property Node" class="XYGraph (strict)"(reference=w424, error in=w425, "Active Cursor"=u32 0, "Cursor.Cursor X"=w423) -> (error out=w422:errorcluster)  [unwired: 1 out]
            n160 = Build Array (concatenate)(w420, "MACRO - Refresh Lists", "Update Cursor Controls") -> (w419:string[])
            n161 = Bundle By Name(cluster=w427, "Rem List"=w417, "Add List"=w417) -> (w418:T2)
          }
          event "Edges Removed": Value Change {
            n162 = event-data() -> ("NewVal"=w429:i32)  [unwired: 1 in]
            n163 = Build Array (concatenate)(w435, "MACRO - Refresh Lists") -> (w434:string[])
            n164 = Bundle By Name(cluster=w432, "Rem List"=w429, "Add List"=-1) -> (w430:T2)
          }
          event "Pulses Added": Value Change {
            n165 = event-data() -> ("NewVal"=w436:i32)  [unwired: 1 in]
            n166 = Bundle By Name(cluster=w440, "Rem List"=-1 ("Add List"), "Add List"=w436) -> (w438:T2)
            n167 = Build Array (concatenate)(w443, "MACRO - Refresh Lists") -> (w442:string[])
          }
          event "remove_remove": Value Change {
            n168 = event-data() -> ()  [unwired: 1 in, 2 out]
            n169 = Unbundle By Name(w461) -> ("Patterns"=w453:T3[], "Sel patterns"=w460:i32[], "Rem List"=w450:i32)
            n170 = Index Array(array=w460) -> (element=w452:i32)  [unwired: 1 in]
            n171 = Index Array(array=w453, index=w452) -> (element=w451:T3)
            n172 = Unbundle By Name(w451) -> ("Remove"=w455:T5[])
            n173 = Delete From Array(array=w455, index=w450) -> (array with subset deleted=w459:T5[])  [unwired: 1 in, 1 out]
            n174 = Build Array (concatenate)(w463, string[] ["Refresh Remove List", "Update Pattern Controls", "MACRO - Refresh Patterns"]) -> (w446:string[])
            n175 = Array Size(array=w459) -> (size(s)=w456:i32)
            n176 = Bundle By Name(cluster=w451, "Remove"=w459) -> (w454:T3)
            n177 = Decrement(x=w456) -> (x-1=w457:i32)
            n178 = In Range and Coerce(upper limit=w457, x=w450, lower limit=-1) -> (coerced(x)=w447:i32)  [unwired: 1 out]
            n179 = Replace Array Subset(array=w453, new element=w454, index=w452) -> (w448:T3[])
            n180 = Bundle By Name(cluster=w461, "Patterns"=w448, "Rem List"=w447, "Need save"=TRUE) -> (w449:T2)
          }
          event "add_remove": Value Change {
            n181 = event-data() -> ()  [unwired: 1 in, 2 out]
            n182 = Unbundle By Name(w481) -> ("Patterns"=w473:T3[], "Sel patterns"=w480:i32[], "Add List"=w470:i32)
            n183 = Index Array(array=w480) -> (element=w472:i32)  [unwired: 1 in]
            n184 = Index Array(array=w473, index=w472) -> (element=w471:T3)
            n185 = Unbundle By Name(w471) -> ("Add"=w475:T6[])
            n186 = Delete From Array(array=w475, index=w470) -> (array with subset deleted=w479:T6[])  [unwired: 1 in, 1 out]
            n187 = Build Array (concatenate)(w483, string[] ["Refresh Add List", "Update Pattern Controls", "MACRO - Refresh Patterns"]) -> (w466:string[])
            n188 = Array Size(array=w479) -> (size(s)=w476:i32)
            n189 = Bundle By Name(cluster=w471, "Add"=w479) -> (w474:T3)
            n190 = Decrement(x=w476) -> (x-1=w477:i32)
            n191 = In Range and Coerce(upper limit=w477, x=w470, lower limit=-1) -> (coerced(x)=w467:i32)  [unwired: 1 out]
            n192 = Replace Array Subset(array=w473, new element=w474, index=w472) -> (w468:T3[])
            n193 = Bundle By Name(cluster=w481, "Patterns"=w468, "Add List"=w467, "Need save"=TRUE) -> (w469:T2)
          }
          event "remove_add": Value Change {
            # "internally teeth are zero indexed, but they are 1 indexed on GUI"
            n194 = event-data() -> ()  [unwired: 1 in, 2 out]
            n195 = Unbundle By Name(w503) -> ("Patterns"=w499:T3[], "Sel patterns"=w502:i32[], "Rem List"=w485:i32)
            n196 = Index Array(array=w502) -> (element=w498:i32)  [unwired: 1 in]
            n197 = Index Array(array=w499, index=w498) -> (element=w497:T3)
            n198 = case shown="0, Default" w485 {
              selector: w485 -> [w511 _]
              tunnel: w497 -> [w512 w519]
              tunnel: [w508 w518] -> w491
              tunnel: [w510 w517] -> w490
              tunnel: [w506 w513] -> w484
              frame 0, Default {
                n199 = Unbundle By Name(w512) -> ("Remove"=w510:T5[])
                n200 = Index Array(array=w510, index=w511) -> (element=w509:T5)
                n201 = Unbundle By Name(w509) -> ("Edge"=w508:bool, "Tooth"=w507:u16)
                n202 = Increment(x=w507) -> (x+1=w506:u16)
              }
              frame -1 {
                n203 = Unbundle By Name(w519) -> ("Remove"=w517:T5[], "Base.Width"=w515:dbl)
                n204 = local read "Chart_Offset"() -> (w516:dbl)
                n205 = local read "Chart_Tooth"() -> (w514:u16)
                n206 = Less?(x=w515, y=w516) -> (x < y?=w518:bool)
                n207 = Decrement(x=w514) -> (x-1=w513:u16)
              }
            }
            n208 = Bundle By Name(cluster=T5 {"Tooth"=0, "Edge"=FALSE} ("Cluster"), "Edge"=w491, "Tooth"=w484) -> (w492:T5)
            n209 = Build Array (concatenate)(w505, string[] ["Refresh Remove List", "Update Pattern Controls", "MACRO - Refresh Patterns"]) -> (w494:string[])
            n210 = Build Array (concatenate)(w490, w492) -> (w489:T5[])
            n211 = Array Size(array=w489) -> (size(s)=w501:i32)
            n212 = Bundle By Name(cluster=w497, "Remove"=w489) -> (w500:T3)
            n213 = Decrement(x=w501) -> (x-1=w488:i32)
            n214 = Replace Array Subset(array=w499, new element=w500, index=w498) -> (w495:T3[])
            n215 = Bundle By Name(cluster=w503, "Patterns"=w495, "Rem List"=w488, "Need save"=TRUE) -> (w496:T2)
          }
          event "add_add": Value Change {
            # "internally teeth are zero indexed, but they are 1 indexed on GUI"
            n216 = event-data() -> ()  [unwired: 1 in, 2 out]
            n217 = Unbundle By Name(w540) -> ("Patterns"=w536:T3[], "Sel patterns"=w539:i32[])
            n218 = Index Array(array=w539) -> (element=w535:i32)  [unwired: 1 in]
            n219 = local read "Chart_Offset"() -> (w522:dbl)
            n220 = local read "Chart_Tooth"() -> (w527:u16)
            n221 = Index Array(array=w536, index=w535) -> (element=w534:T3)
            n222 = Unbundle By Name(w534) -> ("Add"=w528:T6[], "Base.Width"=w523:dbl)
            n223 = Decrement(x=w527) -> (x-1=w520:u16)
            n224 = Bundle By Name(cluster=T6 {"Tooth"=0, "Offset"=0.0, "Width"=0.0} ("Cluster"), "Width"=w523, "Offset"=w522, "Tooth"=w520) -> (w529:T6)
            n225 = Build Array (concatenate)(w528, w529) -> (w526:T6[])
            n226 = Build Array (concatenate)(w542, string[] ["Refresh Add List", "Update Pattern Controls", "MACRO - Refresh Patterns"]) -> (w531:string[])
            n227 = Array Size(array=w526) -> (size(s)=w538:i32)
            n228 = Bundle By Name(cluster=w534, "Add"=w526) -> (w537:T3)
            n229 = Decrement(x=w538) -> (x-1=w525:i32)
            n230 = Replace Array Subset(array=w536, new element=w537, index=w535) -> (w532:T3[])
            n231 = Bundle By Name(cluster=w540, "Patterns"=w532, "Add List"=w525, "Need save"=TRUE) -> (w533:T2)
          }
        }
      }
      frame "Error" {
        n232 = call <vilib>:"Simple Error Handler.vi"("error in (no error)"=w548) -> ()  [unwired: 4 in, 5 out]
        n233 = Unbundle By Name(w546) -> ("Init done"=w545:bool)
        n234 = case shown="True" w545 {
          tunnel: w544 -> [w551 w552]
          tunnel: [w550 w552] -> w543
          frame False {
            n235 = Build Array (concatenate)(string[] ["Release SE Cursor", "MACRO - Shut Down"], w551) -> (w550:string[])
          }
          frame True {
          }
        }
      }
      frame "Set Busy Cursor" {
        n236 = Unbundle By Name(w554) -> ("SE ref"=w553:refnum<vi>)
        n237 = call <vilib>:"Set Busy.vi"("error in (no error)"=w556, "VI reference (current VI)"=w553) -> ("error out"=w555:errorcluster)  [unwired: 8 in, 1 out]
      }
      frame "Clear Busy Cursor" {
        n238 = Unbundle By Name(w559) -> ("SE ref"=w558:refnum<vi>)
        n239 = call <vilib>:"Unset Busy.vi"("VI reference (current VI)"=w558) -> ()  [unwired: 10 in, 1 out]
      }
      frame "<------------- Front Panel Updates------------->" {
      }
      frame "Disable Add and Remove" {
        n240 = Unbundle By Name(w570) -> ("Ctrl Refs.Add List"=w568:refnum<vi>, "Ctrl Refs.Remove List"=w569:refnum<vi>, "Ctrl Refs.remove_add"=w579:refnum<vi>, "Ctrl Refs.remove_remove"=w578:refnum<vi>, "Ctrl Refs.add_remove"=w577:refnum<vi>, "Ctrl Refs.add_Tooth"=w576:refnum<vi>, "Ctrl Refs.add_Width"=w575:refnum<vi>, "Ctrl Refs.add_Offset"=w574:refnum<vi>, "Ctrl Refs.remove_Tooth"=w573:refnum<vi>, "Ctrl Refs.remove_Edge"=w572:refnum<vi>, "Ctrl Refs.add_add"=w565:refnum<vi>)
        n241 = Build Array(w568, w569, w579, w578, w577, w576, w575, w574, w573, w572, w565) -> (w566:refnum<vi>[])
        n242 = call "Enable_Disable Controls.vi"("Enable?"=FALSE ("Enabled?"), "Controls"=w566) -> ()  [unwired: 10 in]
      }
      frame "Plot Pattern(s)" {
        n243 = Unbundle By Name(w586) -> ("Ctrl Refs.Zoom"=w585:refnum<vi>, "Ctrl Refs.Pattern Plot"=w584:refnum<vi>, "Patterns"=w583:T3[], "rotations"=w582:u16, "Sel patterns"=w581:i32[])
        n244 = call "Expand Digital Pattern.vi"("Zoom"=w585, "Pattern Plot"=w584, "error in (no error)"=w588, "Select Patterns"=w581, "Rotations"=w582, "Patterns"=w583) -> ("error out"=w587:errorcluster)  [unwired: 5 in]
      }
      frame "Update Pattern Controls" {
        n245 = call "Update Digital Pattern Pattern Controls.vi"("error in (no error)"=w593, "Page Data in"=w590) -> ("error out"=w592:errorcluster)  [unwired: 9 in]
        n246 = call "Update Digital Pattern FPGA Resources.vi"("error in (no error)"=w592, "Page Data in"=w590) -> ("error out"=w591:errorcluster)  [unwired: 9 in]
      }
      frame "Update Cursor Controls" {
        n247 = call "Update Digital Pattern Cursor Controls.vi"("error in (no error)"=w597, "Page Data in"=w595) -> ("error out"=w596:errorcluster)  [unwired: 9 in]
      }
      frame "Populate Patterns List" {
        n248 = Unbundle By Name(w607) -> ("Patterns"=w605:T3[], "Sel patterns"=w604:i32[], "Ctrl Refs.Select Pattern"=w602:refnum<vi>)
        n249 = for {
          tunnel: w605 -> [w616] mode=indexing
          tunnel: [w615] -> w601 mode=indexing
          n250 = Unbundle By Name(w616) -> ("Name"=w615:string)
        }
        n251 = Array Size(array=w601) -> (size(s)=w606:i32)
        n252 = for {
          tunnel: w606 -> [w614]
          tunnel: [w612] -> w599 mode=indexing if=w610
          tunnel: w604 -> [w611] mode=indexing
          n253 = In Range and Coerce(upper limit=w614, x=w611, lower limit=0) -> (coerced(x)=w612:i32, In Range?=w610:bool)
        }
        n254 = property class="LstBox (strict)"(reference=w602, error in=w608, "Item Names"=w601, "Value"=w599) -> (error out=w603:errorcluster)  [unwired: 1 out]
        n255 = Bundle By Name(cluster=w607, "Sel patterns"=w599) -> (w600:T2)
      }
      frame "Set Remove Available" {
        n256 = Unbundle By Name(w625) -> ("Ctrl Refs.remove_add"=w620:refnum<vi>, "Ctrl Refs.remove_remove"=w624:refnum<vi>, "Ctrl Refs.remove_Tooth"=w622:refnum<vi>, "Ctrl Refs.remove_Edge"=w621:refnum<vi>)
        n257 = Build Array(w620) -> (w619:refnum<vi>[])
        n258 = Build Array(w624, w622, w621) -> (w623:refnum<vi>[])
        n259 = call "Enable_Disable Controls.vi"("Enable?"=TRUE, "Controls"=w619) -> ()  [unwired: 10 in]
        n260 = call "Enable_Disable Controls.vi"("Enable?"=FALSE, "Controls"=w623) -> ()  [unwired: 10 in]
      }
      frame "Set Remove Unavailable" {
        n261 = Unbundle By Name(w636) -> ("Ctrl Refs.remove_add"=w631:refnum<vi>, "Ctrl Refs.remove_remove"=w635:refnum<vi>, "Ctrl Refs.remove_Tooth"=w633:refnum<vi>, "Ctrl Refs.remove_Edge"=w632:refnum<vi>)
        n262 = Build Array(w631) -> (w630:refnum<vi>[])
        n263 = Build Array(w635, w633, w632) -> (w634:refnum<vi>[])
        n264 = call "Enable_Disable Controls.vi"("Enable?"=TRUE, "Controls"=w630) -> ()  [unwired: 10 in]
        n265 = call "Enable_Disable Controls.vi"("Enable?"=TRUE, "Controls"=w634) -> ()  [unwired: 10 in]
      }
      frame "Set Add Available" {
        n266 = Unbundle By Name(w648) -> ("Ctrl Refs.add_add"=w643:refnum<vi>, "Ctrl Refs.add_remove"=w647:refnum<vi>, "Ctrl Refs.add_Tooth"=w645:refnum<vi>, "Ctrl Refs.add_Width"=w644:refnum<vi>, "Ctrl Refs.add_Offset"=w640:refnum<vi>)
        n267 = Build Array(w643) -> (w642:refnum<vi>[])
        n268 = Build Array(w647, w645, w644, w640) -> (w646:refnum<vi>[])
        n269 = call "Enable_Disable Controls.vi"("Enable?"=TRUE, "Controls"=w642) -> ()  [unwired: 10 in]
        n270 = call "Enable_Disable Controls.vi"("Enable?"=FALSE, "Controls"=w646) -> ()  [unwired: 10 in]
      }
      frame "Set Add Unavailable" {
        n271 = Unbundle By Name(w660) -> ("Ctrl Refs.add_add"=w655:refnum<vi>, "Ctrl Refs.add_remove"=w659:refnum<vi>, "Ctrl Refs.add_Tooth"=w657:refnum<vi>, "Ctrl Refs.add_Width"=w656:refnum<vi>, "Ctrl Refs.add_Offset"=w652:refnum<vi>)
        n272 = Build Array(w655) -> (w654:refnum<vi>[])
        n273 = Build Array(w659, w657, w656, w652) -> (w658:refnum<vi>[])
        n274 = call "Enable_Disable Controls.vi"("Enable?"=TRUE, "Controls"=w654) -> ()  [unwired: 10 in]
        n275 = call "Enable_Disable Controls.vi"("Enable?"=TRUE, "Controls"=w658) -> ()  [unwired: 10 in]
      }
      frame "Refresh Add List" {
        n276 = Unbundle By Name(w667) -> ("Patterns"=w672:T3[], "Sel patterns"=w671:i32[], "Ctrl Refs.Pattern Plot"=w670:refnum<vi>, "Add List"=w664:i32, "rotations"=w663:u16)
        n277 = case shown="Default" w664 {
          selector: w664 -> [_ w679]
          tunnel: w672 -> [_ w699]
          tunnel: w671 -> [_ w698]
          tunnel: w670 -> [_ w684]
          tunnel: w669 -> [w675 w681]
          tunnel: [w675 w680] -> w668
          tunnel: [string[] ["Set Add Available"] string[] ["Set Add Unavailable", "Update Cursor Controls"]] -> w665
          tunnel: w663 -> [_ w678]
          frame -1 {
          }
          frame Default {
            # "internally teeth are zero indexed, but they are 1 indexed on GUI"
            n278 = Index Array(array=w698) -> (element=w697:i32)  [unwired: 1 in]
            n279 = Index Array(array=w699, index=w697) -> (element=w696:T3)
            n280 = Unbundle By Name(w696) -> ("Add"=w695:T6[], "Base.Length"=w691:dbl, "Base.Teeth"=w690:u16, "Base.Offset"=w689:dbl)
            n281 = Index Array(array=w695, index=w679) -> (element=w694:T6)
            n282 = Unbundle By Name(w694) -> ("Tooth"=w688:u16, "Offset"=w683:dbl, "Width"=w682:dbl)
            n283 = Divide(x=w691, y=w690) -> (x/y=w693:dbl)
            n284 = Multiply(x=w688, y=w693) -> (x*y=w692:dbl)
            n285 = Increment(x=w688) -> (x+1=w676:u16)
            n286 = Compound Arithmetic op=ADD(w692, w683, w689) -> (w687:dbl)
            n287 = local write "add_Offset"(w683) -> ()
            n288 = local write "add_Tooth"(w676) -> ()
            n289 = call "Digital Pattern Wrap Around.vi"("Rotations"=w678, "x"=w687) -> ("x"=w685:dbl)  [unwired: 9 in]
            n290 = local write "add_Width"(w682) -> ()
            n291 = property on="Property Node" class="XYGraph (strict)"(reference=w684, error in=w681, "Active Cursor"=u32 0, "Cursor.Cursor X"=w685) -> (error out=w680:errorcluster)  [unwired: 1 out]
          }
        }
        n292 = local write "Pulses Added"(w664) -> ()
        n293 = Build Array (concatenate)(w665, w673) -> (w666:string[])
      }
      frame "Refresh Remove List" {
        n294 = Unbundle By Name(w700) -> ("Rem List"=w701:i32)
        n295 = case shown="Default" w701 {
          selector: w701 -> [_ w713]
          tunnel: w705 -> [w708 w715]
          tunnel: [w708 w714] -> w704
          tunnel: [string[] ["Set Remove Available"] string[] ["Set Remove Unavailable", "Update Cursor Controls"]] -> w702
          tunnel: w700 -> [_ w712]
          frame -1 {
          }
          frame Default {
            # "internally teeth are zero indexed, but they are 1 indexed on GUI"
            n296 = Unbundle By Name(w712) -> ("Patterns"=w735:T3[], "Sel patterns"=w734:i32[], "Ctrl Refs.Pattern Plot"=w716:refnum<vi>, "rotations"=w711:u16)
            n297 = Index Array(array=w734) -> (element=w733:i32)  [unwired: 1 in]
            n298 = Index Array(array=w735, index=w733) -> (element=w732:T3)
            n299 = Unbundle By Name(w732) -> ("Base.Width"=w724:dbl, "Remove"=w731:T5[], "Base.Length"=w723:dbl, "Base.Teeth"=w722:u16, "Base.Offset"=w721:dbl)
            n300 = Index Array(array=w731, index=w713) -> (element=w730:T5)
            n301 = Unbundle By Name(w730) -> ("Tooth"=w720:u16, "Edge"=w725:bool)
            n302 = Increment(x=w720) -> (x+1=w709:u16)
            n303 = Select(t=w724, s=w725, f=sgl 0.0) -> (s? t:f=w729:dbl)
            n304 = local write "remove_Tooth"(w709) -> ()
            n305 = Divide(x=w723, y=w722) -> (x/y=w728:dbl)
            n306 = local write "Edge"(w725) -> ()
            n307 = Multiply(x=w720, y=w728) -> (x*y=w727:dbl)
            n308 = Compound Arithmetic op=ADD(w727, w729, w721) -> (w719:dbl)
            n309 = call "Digital Pattern Wrap Around.vi"("Rotations"=w711, "x"=w719) -> ("x"=w717:dbl)  [unwired: 9 in]
            n310 = property on="Property Node" class="XYGraph (strict)"(reference=w716, error in=w715, "Active Cursor"=u32 0, "Cursor.Cursor X"=w717) -> (error out=w714:errorcluster)  [unwired: 1 out]
          }
        }
        n311 = local write "Edges Removed"(w701) -> ()
        n312 = Build Array (concatenate)(w702, w706) -> (w703:string[])
      }
      frame "Hide Cursors and Edit Controls" {
        n313 = Unbundle By Name(w758) -> ("Ctrl Refs.Add List"=w757:refnum<vi>, "Ctrl Refs.Remove List"=w756:refnum<vi>, "Ctrl Refs.Pattern Name"=w755:refnum<vi>, "Ctrl Refs.remove_add"=w754:refnum<vi>, "Ctrl Refs.remove_remove"=w753:refnum<vi>, "Ctrl Refs.add_remove"=w752:refnum<vi>, "Ctrl Refs.base_Length"=w751:refnum<vi>, "Ctrl Refs.base_teeth"=w750:refnum<vi>, "Ctrl Refs.base_Toothwidth"=w749:refnum<vi>, "Ctrl Refs.base_Offset"=w748:refnum<vi>, "Ctrl Refs.add_Tooth"=w747:refnum<vi>, "Ctrl Refs.add_Width"=w746:refnum<vi>, "Ctrl Refs.add_Offset"=w745:refnum<vi>, "Ctrl Refs.remove_Tooth"=w744:refnum<vi>, "Ctrl Refs.remove_Edge"=w743:refnum<vi>, "Ctrl Refs.Chart_Position"=w742:refnum<vi>, "Ctrl Refs.Chart_Tooth"=w741:refnum<vi>, "Ctrl Refs.Chart_Offset"=w740:refnum<vi>, "Ctrl Refs.add_add"=w739:refnum<vi>, "Ctrl Refs.FPGA Resource"=w738:refnum<vi>)
        n314 = Build Array(w757, w756, w755, w754, w753, w752, w751, w750, w749, w748, w747, w746, w745, w744, w743, w742, w741, w740, w739, w738) -> (w737:refnum<vi>[])
        n315 = call "Hide_Show Controls.vi"("Hide?"=TRUE, "Controls"=w737) -> ()  [unwired: 10 in]
      }
      frame "Show Cursors and Edit Controls" {
        n316 = Unbundle By Name(w783) -> ("Ctrl Refs.Add List"=w782:refnum<vi>, "Ctrl Refs.Remove List"=w781:refnum<vi>, "Ctrl Refs.Pattern Name"=w780:refnum<vi>, "Ctrl Refs.remove_add"=w779:refnum<vi>, "Ctrl Refs.remove_remove"=w778:refnum<vi>, "Ctrl Refs.add_remove"=w777:refnum<vi>, "Ctrl Refs.base_Length"=w776:refnum<vi>, "Ctrl Refs.base_teeth"=w775:refnum<vi>, "Ctrl Refs.base_Toothwidth"=w774:refnum<vi>, "Ctrl Refs.base_Offset"=w773:refnum<vi>, "Ctrl Refs.add_Tooth"=w772:refnum<vi>, "Ctrl Refs.add_Width"=w771:refnum<vi>, "Ctrl Refs.add_Offset"=w770:refnum<vi>, "Ctrl Refs.remove_Tooth"=w769:refnum<vi>, "Ctrl Refs.remove_Edge"=w768:refnum<vi>, "Ctrl Refs.Chart_Position"=w767:refnum<vi>, "Ctrl Refs.Chart_Tooth"=w766:refnum<vi>, "Ctrl Refs.Chart_Offset"=w765:refnum<vi>, "Ctrl Refs.add_add"=w764:refnum<vi>, "Ctrl Refs.FPGA Resource"=w763:refnum<vi>)
        n317 = Build Array(w782, w781, w780, w779, w778, w777, w776, w775, w774, w773, w772, w771, w770, w769, w768, w767, w766, w765, w764, w763) -> (w762:refnum<vi>[])
        n318 = call "Hide_Show Controls.vi"("Hide?"=FALSE, "Controls"=w762) -> ()  [unwired: 10 in]
      }
      frame "Add Remove Pattern EnableDisable" {
        n319 = Unbundle By Name(w798) -> ("Patterns"=w797:T3[], "FPGA Resources"=w796:string[], "Ctrl Refs.pattern_add"=w794:refnum<vi>, "Ctrl Refs.pattern_remove"=w789:refnum<vi>)
        n320 = Array Size(array=w797) -> (size(s)=w790:i32)
        n321 = Array Size(array=w796) -> (size(s)=w795:i32)
        n322 = Greater Or Equal?(x=w790, y=w795) -> (x >= y?=w792:bool)
        n323 = Build Array(w794) -> (w793:refnum<vi>[])
        n324 = Build Array(w789) -> (w788:refnum<vi>[])
        n325 = Not(x=w792) -> (.not. x?=w791:bool)
        n326 = Equal To 0?(x=w790) -> (x = 0?=w787:bool)
        n327 = call "Enable_Disable Controls.vi"("Enable?"=w791, "Controls"=w793) -> ()  [unwired: 10 in]
        n328 = Not(x=w787) -> (.not. x?=w786:bool)
        n329 = call "Enable_Disable Controls.vi"("Enable?"=w786, "Controls"=w788) -> ()  [unwired: 10 in]
      }
      frame "<------------------ Shut Down ------------------>" {
      }
      frame "Save If Needed" {
        n330 = Unbundle By Name(w808) -> ("Need save"=w804:bool, "Node Ptr"=w806:T1, "Patterns"=w805:T3[])
        n331 = case shown="True" w804 {
          tunnel: w809 -> [w811 w815]
          tunnel: [w811 w814] -> w807
          tunnel: w806 -> [_ w813]
          tunnel: w805 -> [_ w812]
          frame False {
          }
          frame True {
            n332 = call "Save Digital Patterns.vi"("error in (no error)"=w815, "Patterns"=w812, "Item Ref in"=w813) -> ("error out"=w814:errorcluster)  [unwired: 8 in]
          }
        }
      }
      frame "SE Cleanup" {
        n333 = Unbundle By Name(w825) -> ("SE ref"=w819:refnum<vi>, "SysExp Event"=w824:refnum<event-registration>)
        n334 = Unregister For Events(event registration refnum=w824, error in=w821) -> (error out=w823:errorcluster)
        n335 = Close Reference(reference=w819, error in (no error)=w823) -> (error out=w820:errorcluster)
        n336 = invoke class="VI" method="FP.Close"(error in=w820) -> (error out=w817:errorcluster)  [unwired: 2 in, 2 out]
        n337 = call <vilib>:"Clear Errors.vi"("error in (no error)"=w817, "specific error code to clear (0: all)"=1149) -> ("error out"=w816:errorcluster)  [unwired: 4 in, 1 out]
        n338 = call <vilib>:"NI VeriStand - Signal When Ready for Shutdown.vi"("error in (no error)"=w816) -> ("error out"=w822:errorcluster)  [unwired: 10 out]
      }
      frame "Exit" {
      }
      frame "<------------------ Macros ------------------>" {
      }
      frame "MACRO - Initialize" {
        n339 = Build Array (concatenate)(string[] ["Get SE Ref", "Get SE Event Ref", "Get Control References", "Hide Cursors and Edit Controls", "Get Persistent Data", "Get Rotations", "Select All Patterns", "Get Available FPGA Resources", "Add Remove Pattern EnableDisable", "MACRO - Refresh Patterns", "Initialize Pattern Editing", "MACRO - Refresh Lists", "Update Cursor Controls", "Release SE Cursor", "Set Init Done"], w835) -> (w834:string[])
      }
      frame "MACRO - Shut Down" {
        n340 = Build Array (concatenate)(string[] ["Save If Needed", "SE Cleanup", "Clear Busy Cursor", "Exit"], w842) -> (w841:string[])
      }
      frame "MACRO - Refresh Patterns" {
        n341 = Build Array (concatenate)(string[] ["Set Busy Cursor", "Populate Patterns List", "Plot Pattern(s)", "Clear Busy Cursor"], w847) -> (w846:string[])
      }
      frame "MACRO - Refresh Lists" {
        n342 = Build Array (concatenate)(string[] ["Refresh Remove List", "Refresh Add List"], w852) -> (w851:string[])
      }
      frame "<------------------ Initialization ------------------>" {
      }
      frame "Get Control References" {
        n343 = control-ref of="Pattern Plot"() -> (w881:refnum<vi>)
        n344 = control-ref of="remove_add"() -> (w875:refnum<vi>)
        n345 = control-ref of="remove_remove"() -> (w874:refnum<vi>)
        n346 = control-ref of="add_remove"() -> (w873:refnum<vi>)
        n347 = control-ref of="Edge"() -> (w865:refnum<vi>)
        n348 = control-ref of="add_add"() -> (w861:refnum<vi>)
        n349 = control-ref of="pattern_remove"() -> (w860:refnum<vi>)
        n350 = control-ref of="pattern_add"() -> (w859:refnum<vi>)
        n351 = control-ref of="Patterns"() -> (w879:refnum<vi>)
        n352 = control-ref of="Pulses Added"() -> (w878:refnum<vi>)
        n353 = control-ref of="Edges Removed"() -> (w877:refnum<vi>)
        n354 = control-ref of="Header"() -> (w882:refnum<vi>)
        n355 = control-ref of="base_Length"() -> (w872:refnum<vi>)
        n356 = control-ref of="base_teeth"() -> (w857:refnum<vi>)
        n357 = control-ref of="base_Toothwidth"() -> (w871:refnum<vi>)
        n358 = control-ref of="base_Offset"() -> (w870:refnum<vi>)
        n359 = control-ref of="add_Tooth"() -> (w869:refnum<vi>)
        n360 = control-ref of="add_Width"() -> (w868:refnum<vi>)
        n361 = control-ref of="add_Offset"() -> (w867:refnum<vi>)
        n362 = control-ref of="remove_Tooth"() -> (w866:refnum<vi>)
        n363 = control-ref of="Chart_Position"() -> (w864:refnum<vi>)
        n364 = control-ref of="Chart_Tooth"() -> (w863:refnum<vi>)
        n365 = control-ref of="Chart_Offset"() -> (w862:refnum<vi>)
        n366 = control-ref of="Pattern Name"() -> (w876:refnum<vi>)
        n367 = control-ref of="Zoom"() -> (w880:refnum<vi>)
        n368 = control-ref of="FPGA Resource"() -> (w858:refnum<vi>)
        n369 = Bundle By Name(cluster=w886, "Ctrl Refs.Header"=w882, "Ctrl Refs.Pattern Plot"=w881, "Ctrl Refs.Zoom"=w880, "Ctrl Refs.Select Pattern"=w879, "Ctrl Refs.Add List"=w878, "Ctrl Refs.Remove List"=w877, "Ctrl Refs.Pattern Name"=w876, "Ctrl Refs.remove_add"=w875, "Ctrl Refs.remove_remove"=w874, "Ctrl Refs.add_remove"=w873, "Ctrl Refs.base_Length"=w872, "Ctrl Refs.base_teeth"=w857, "Ctrl Refs.base_Toothwidth"=w871, "Ctrl Refs.base_Offset"=w870, "Ctrl Refs.add_Tooth"=w869, "Ctrl Refs.add_Width"=w868, "Ctrl Refs.add_Offset"=w867, "Ctrl Refs.remove_Tooth"=w866, "Ctrl Refs.remove_Edge"=w865, "Ctrl Refs.Chart_Position"=w864, "Ctrl Refs.Chart_Tooth"=w863, "Ctrl Refs.Chart_Offset"=w862, "Ctrl Refs.add_add"=w861, "Ctrl Refs.pattern_remove"=w860, "Ctrl Refs.pattern_add"=w859, "Ctrl Refs.FPGA Resource"=w858) -> (w885:T2)
      }
      frame "Release SE Cursor" {
        n370 = call <vilib>:"NI VeriStand - Unset Busy Cursor.vi"("error in (no error)"=w888) -> ("error out"=w887:errorcluster)  [unwired: 10 out]
      }
      frame "Get SE Event Ref" {
        n371 = call <vilib>:"NI VeriStand - Get Event Refnum.vi"("error in (no error)"=w895) -> ("error out"=w896:errorcluster, "Event Ref"=w897:refnum<user-event>)  [unwired: 9 out]
        n372 = register-events(error in=w896, w897) -> (reference out=w892:refnum<event-registration>, error out=w894:errorcluster)  [unwired: 1 in]
        n373 = Bundle By Name(cluster=w893, "SysExp Event"=w892) -> (w891:T2)
      }
      frame "Get SE Ref" {
        n374 = Open VI Reference(vi path="System Explorer.lvlib:System Explorer.vi" ("Separator (,)"), error in (no error)=w902) -> (vi reference=w899:refnum<vi>, error out=w901:errorcluster)  [unwired: 4 in]
        n375 = Bundle By Name(cluster=w904, "SE ref"=w899) -> (w900:T2)
      }
      frame "Set Init Done" {
        n376 = Bundle By Name(cluster=w908, "Init done"=TRUE) -> (w907:T2)
      }
      frame "Get Persistent Data" {
        n377 = Unbundle By Name(w915) -> ("Node Ptr"=w914:T1)
        n378 = call "Get Digital Patterns - Multi FPGA.vi"("error in (no error)"=w916, "Item Ref in"=w914) -> ("error out"=w912:errorcluster, "Patterns"=w911:T3[])  [unwired: 7 in, 1 out]
        n379 = Bundle By Name(cluster=w915, "Patterns"=w911) -> (w913:T2)
      }
      frame "Get Rotations" {
        n380 = Unbundle By Name(w931) -> ("Ctrl Refs.Zoom"=w924:refnum<vi>, "Node Ptr"=w919:T1)
        n381 = call "Get APU Characteristics.vi"("error in (no error)"=w932, "Item Ref in"=w919) -> ("error out"=w920:errorcluster, "rotations"=w918:u16)  [unwired: 3 in, 5 out]
        n382 = Bundle By Name(cluster=w931, "rotations"=w918) -> (w930:T2)
        n383 = Multiply(x=w918, y=180.0 ("t")) -> (x*y=w928:dbl)
        n384 = Negate(x=w928) -> (-x=w929:dbl)
        n385 = property on="Property Node" class="Slide (strict)"(reference=w924, error in=w920, "Scale.Maximum"=w928, "Maximum"=w928, "Minimum"=w929, "Scale.Minimum"=w929) -> (reference out=w923:refnum<vi>, error out=w922:errorcluster, "Value"=w926:cluster{dbl, dbl})
        n386 = Bundle(cluster=w926, w928, w929) -> (w927:cluster{dbl, dbl})
        n387 = property on="Property Node" class="Slide (strict)"(reference=w923, error in=w922, "Val(Sgnl)"=w927) -> (error out=w921:errorcluster)  [unwired: 1 out]
      }
      frame "Get Available FPGA Resources" {
        n388 = Unbundle By Name(w945) -> ("Ctrl Refs.FPGA Resource"=w942:refnum<vi>, "Node Ptr"=w937:T1)
        n389 = global read "Properties.vi" "Main.Digital PatGens"() -> (w936:string)
        n390 = global read "Constants and GUIDs.vi" "Constant.Pick FPGA resource"() -> (w941:string)
        n391 = call "Get Channels For Measurement.vi"("error in (no error)"=w938, "property name"=w936, "Node Ptr in"=w937) -> ("error out"=w935:errorcluster, "rios and channels"=w934:T12)  [unwired: 6 in, 1 out]
        n392 = for {
          tunnel: w934 -> [w948] mode=indexing
          tunnel: [w947] -> w939 mode=concatenating
          n393 = Unbundle(w948) -> (w947:string[])  [unwired: 1 out]
        }
        n394 = Build Array (concatenate)(w941, w939) -> (w940:string[])
        n395 = Bundle By Name(cluster=w945, "FPGA Resources"=w939) -> (w944:T2)
        n396 = property class="Ring (strict)"(reference=w942, error in=w935, "Strings []"=w940) -> (error out=w943:errorcluster)  [unwired: 1 out]
      }
      frame "Select All Patterns" {
        n397 = Unbundle By Name(w953) -> ("Patterns"=w952:T3[])
        n398 = Array Size(array=w952) -> (size(s)=w950:i32)
        n399 = for {
          N: w950 -> [_]
          tunnel: [w956] -> w949 mode=indexing
          i -> [w956]
        }
        n400 = Bundle By Name(cluster=w953, "Sel patterns"=w949) -> (w951:T2)
      }
      frame "Initialize Pattern Editing" {
        n401 = Unbundle By Name(w958) -> ("Sel patterns"=w962:i32[])
        n402 = Array Size(array=w962) -> (size(s)=w959:i32)
        n403 = case shown="1" w959 {
          tunnel: w961 -> [w965 w968]
          tunnel: [w964 w967] -> w960
          frame 1 {
            n404 = Build Array (concatenate)(string[] ["Update Pattern Controls", "Show Cursors and Edit Controls"], w965) -> (w964:string[])
          }
          frame Default {
            n405 = Build Array (concatenate)(string[] ["Hide Cursors and Edit Controls"], w968) -> (w967:string[])
          }
        }
      }
    }
    n406 = case shown="Error" w10 {
      tunnel: w15 -> [w19 w20]
      tunnel: [w19 w21] -> w13
      frame No Error {
      }
      frame Error {
        n407 = Build Array (concatenate)("Error", w20) -> (w21:string[])
      }
    }
  }
  "error out" <- w5
